vi "PlungeMap_nano.vi"(10 "Scaling?":bool, 11 "Input (pA)":dbl) -> (3 "output":dbl)   [LabVIEW 2019]
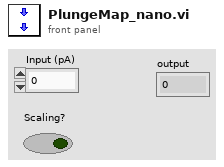
[diagram p1: front panel]
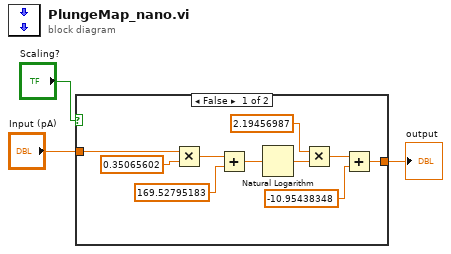
[diagram p0: block diagram]
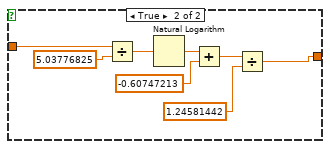
[diagram p2: hidden frame]
diagram:
  n1 = case shown="False" "Scaling?" {
    tunnel: "Input (pA)" -> [w5 w21]
    tunnel: [w4 w16] -> w2
    frame False {
      n2 = Multiply(x=w5, y=0.35065602) -> (x*y=w12:dbl)
      n3 = Add(x=w12, y=169.52795183) -> (x+y=w10:dbl)
      n4 = Natural Logarithm(1:w10) -> (0:w9:dbl)
      n5 = Multiply(x=2.19456987, y=w9) -> (x*y=w7:dbl)
      n6 = Add(x=w7, y=-10.95438348) -> (x+y=w4:dbl)
    }
    frame True {
      n7 = Divide(x=w21, y=5.03776825) -> (x/y=w19:dbl)
      n8 = Natural Logarithm(1:w19) -> (0:w18:dbl)
      n9 = Add(x=w18, y=-0.60747213) -> (x+y=w17:dbl)
      n10 = Divide(x=w17, y=1.24581442) -> (x/y=w16:dbl)
    }
  }
  "output" <- w2
